vi "interweave_vector.vi"(6 "element (0)":dbl, 9 "indices w.r.t. list":i32[](array[numeric]), 10 "vector in":dbl[](array[numeric])) -> (1 "indices w.r.t. list out":i32[](array[numeric]), 2 "vector out":dbl[](array[numeric]))   [LabVIEW 2015]
panel:
  out "index of element":i32
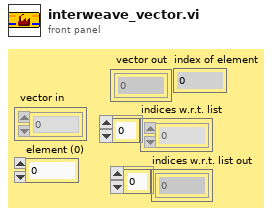
[diagram p1: front panel]
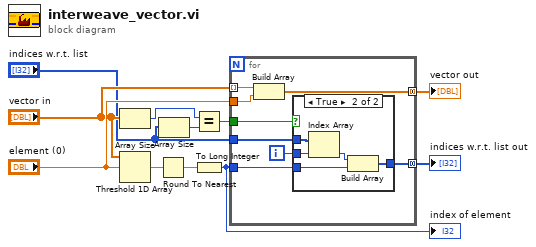
[diagram p0: block diagram]
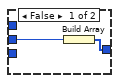
[diagram p2: hidden frame]
diagram:
  n1 = Array Size(array="vector in") -> (size(s)=w3:i32)
  n2 = Threshold 1D Array(2:"element (0)", 3:"vector in") -> (0:w10:dbl)  [unwired: 1 in]
  n3 = Round To Nearest(number=w10) -> (nearest integer value=w9:dbl)
  n4 = Array Size(array="indices w.r.t. list") -> (size(s)=w2:i32)
  n5 = Equal?(x=w3, y=w2) -> (x = y?=w1:bool)
  n6 = To Long Integer(number=w9) -> (32bit integer=w8:i32)
  "index of element" <- w8
  n7 = for {
    tunnel: "vector in" -> [w19] mode=indexing
    tunnel: "indices w.r.t. list" -> [w14]
    tunnel: "element (0)" -> [w18]
    tunnel: [w17] -> w7 mode=concatenating
    tunnel: w8 -> [w16]
    tunnel: [w15] -> w6 mode=concatenating
    tunnel: w1 -> [w12]
    i -> [w13]
    n8 = Build Array(w19, w18) -> (w17:dbl[])
    n9 = case shown="True" w12 {
      tunnel: w16 -> [_ w26]
      tunnel: [w20 w25] -> w15
      tunnel: w14 -> [_ w24]
      tunnel: w13 -> [w21 w22]
      frame False {
        n10 = Build Array(w21) -> (w20:i32[])
      }
      frame True {
        n11 = Index Array(array=w24, index=w22) -> (element=w23:i32)
        n12 = Build Array(w23, w26) -> (w25:i32[])
      }
    }
  }
  "vector out" <- w7
  "indices w.r.t. list out" <- w6
